vi "VisionTrack.vi"(6 "RobotLength (in)":dbl format="%#_13g", 7 "target height(in)":dbl=36.0 format="%#_13g", 8 "error in (no error)":errorcluster, 9 "mounting angle (degrees)":dbl format="%#_13g", 10 "camera height(in)":dbl=8.0, 11 "Vision in":refnum<class "Vision.lvclass">) -> (0 "error out":errorcluster, 1 "VerticalOffset(degrees)":dbl format="%#_13g", 2 "HorizontalOffset(degrees)":dbl, 3 "Vision out":refnum<class "Vision.lvclass">, 4 "Target?":bool, 5 "Distance(in)":dbl format="%#_13g")   [LabVIEW 2018, in "Vision.lvlib" / "Vision.lvclass"]
doc: "tv Whether the limelight has any valid targets (0 or 1)\ntx Horizontal Offset From Crosshair To Target (-27 degrees to 27 degrees)\nty Vertical Offset From Crosshair To Target (-20.5 degrees to 20.5 degrees)\nta Target Area (0% of image to 100% of image)\nts Skew or rotation (-90 degrees to 0 degrees)\ntl The pipeline’s latency contribution (ms) Add at least 11ms for image capture latency.\ntshort Sidelength of shortest side of the fitted bounding box (pixels)\ntlong Sidelength of longest side of the fitted bounding box (pixels)\nthor Horizontal sidelength of the rough bounding box (0 - 320 pixels)\ntvert Vertical sidelength of the rough bounding box (0 - 320 pixels)\ngetpipe True active pipeline index of the camera (0 .. 9)"
uses:
  Vision.lvclass
panel:
  out "average distance(in)":dbl
  # "#TODO\nMake this an outout cluster, instead of\nusing all the connectors in the icon pane"
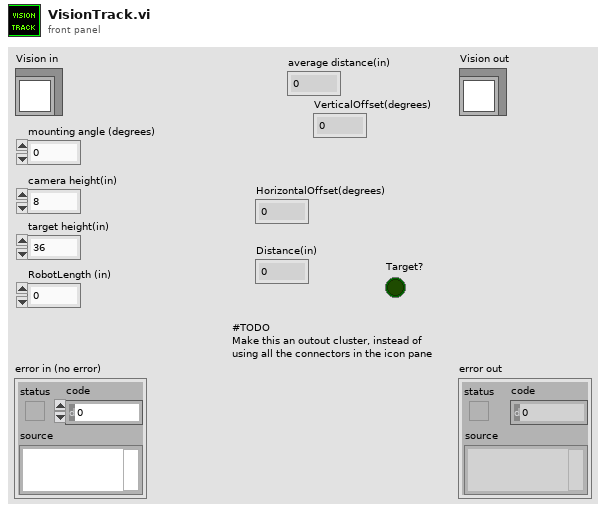
[diagram p1: front panel]
types:
  T1 = typedef "Vision.lvlib/Vision.lvclass/LimeLightData.ctl" = cluster{"Target?(tv)":dbl, "HorOffset(tx)":dbl, "VertOffset(ty)":dbl, "TargetArea(ta)":dbl, "Skew/roll(ts)":dbl, "PipelinLatency(tl)":dbl, "Sidelength of shortest side of the fitted bounding box (tshort) ":dbl, "Sidelength of longest side of the fitted bounding box (tlong)":dbl, "Horizontal sidelength of the rough bounding box (thor)":dbl, "Vertical sidelength of the rough bounding box (tvert)":dbl, "Pipeline?(GetPipe)":dbl, "camtran(x)":dbl, "camtran(y)":dbl, "camtran(z)":dbl, "camtran(pitch)":dbl, "camtran(yaw)":dbl, "camtran(roll)":dbl}
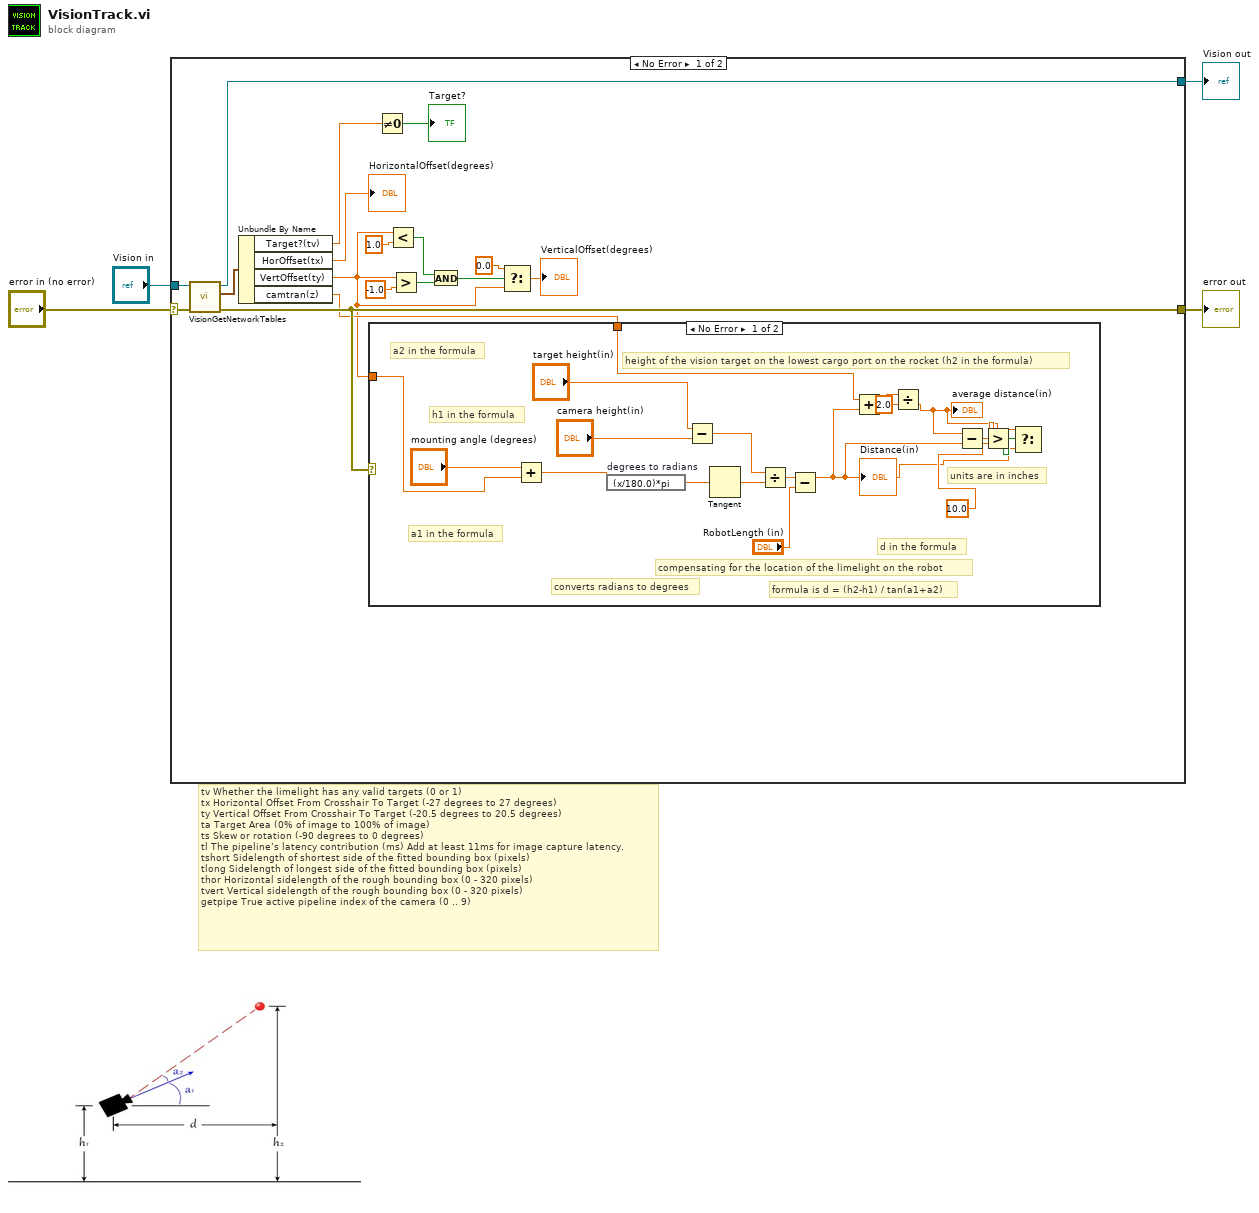
[diagram p0: block diagram]
diagram:
  # "tv\tWhether the limelight has any valid targets (0 or 1)\ntx\tHorizontal Offset From Crosshair To Target (-27 degrees to 27 degrees)\nty\tVertical Offset From Crosshair To Target (-20.5 degrees to 20.5 degrees)\nta\tTarget Area (0% of image to 100% of image)\nts\tSkew or rotation (-90 degrees to 0 degrees)\ntl\tThe pipeline’s latency contribution (ms) Add at least 11ms for image capture latency.\ntshort\tSidelength of shortest side of the fitted bounding box (pixels)\ntlong\tSidelength of longest side of the fitted bounding box (pixels)\nthor\tHorizontal sidelength of the rough bounding box (0 - 320 pixels)\ntvert\tVertical sidelength of the rough bounding box (0 - 320 pixels)\ngetpipe\tTrue active pipeline index of the camera (0 .. 9)"
  n1 = case shown="No Error" "error in (no error)" {
    selector: "error in (no error)" -> [w18 w41]
    tunnel: [w16 w41] -> w3
    tunnel: [w19 w40] -> w1
    tunnel: "Vision in" -> [w21 w40]
    frame No Error {
      n2 = call "VisionGetNetworkTables.vi"("error in (no error)"=w18, "Vision in"=w21) -> ("error out"=w16:errorcluster, "Cluster"=w20:T1, "Vision out"=w19:refnum<class "Vision.lvclass">)  [unwired: 7 in]
      n3 = Unbundle By Name(w20) -> ("Target?(tv)"=w14:dbl, "HorOffset(tx)"=→"HorizontalOffset(degrees)":dbl, "VertOffset(ty)"=w6:dbl, "camtran(z)"=w13:dbl)
      n4 = case shown="No Error" w16 {
        tunnel: w6 -> [w39 _]
        tunnel: w13 -> [w29 _]
        frame No Error {
          # "compensating for the location of the limelight on the robot"
          # "height of the vision target on the lowest cargo port on the rocket (h2 in the formula)"
          # "d in the formula"
          # "a2 in the formula"
          # "a1 in the formula"
          # "h1 in the formula"
          # "formula is d = (h2-h1) / tan(a1+a2)"
          # "units are in inches"
          # "converts radians to degrees"
          n5 = Add(x="mounting angle (degrees)", y=w39) -> (x+y=w31:dbl)
          n6 = expression code="(x/180.0)*pi" "degrees to radians"(w31) -> (w30:dbl)
          n7 = Subtract(x="target height(in)", y="camera height(in)") -> (x-y=w35:dbl)
          n8 = Tangent(1:w30) -> (0:w34:dbl)
          n9 = Divide(x=w35, y=w34) -> (x/y=w33:dbl)
          n10 = Subtract(x=w33, y="RobotLength (in)") -> (x-y=w23:dbl)
          "Distance(in)" <- w23
          n11 = Add(x=w29, y=w23) -> (x+y=w28:dbl)
          n12 = Divide(x=w28, y=2.0) -> (x/y=w22:dbl)
          "average distance(in)" <- w22
          n13 = Subtract(x=w22, y=w23) -> (x-y=w26:dbl)
          n14 = Greater?(x=w26, y=10.0) -> (0:w24:bool)
          n15 = Select(t=w23, s=w24, f=w22) -> ()  [unwired: 1 out]
        }
        frame Error {
        }
      }
      n16 = Not Equal To 0?(x=w14) -> (x != 0?=→"Target?":bool)
      n17 = Less?(x=w6, y=1.0) -> (x < y?=w10:bool)
      n18 = Greater?(x=w6, y=-1.0) -> (0:w9:bool)
      n19 = And(x=w10, y=w9) -> (x .and. y?=w5:bool)
      n20 = Select(t=0.0, s=w5, f=w6) -> (s? t:f=→"VerticalOffset(degrees)":dbl)
    }
    frame Error {
    }
  }
  "error out" <- w3
  "Vision out" <- w1
